vi "Write datatype.vi"(8 "error in (no error)":errorcluster, 10 "datatype":string, 11 "Datatype group in":refnum<class "Datatype group.lvclass">) -> (0 "error out":errorcluster, 3 "Datatype group out":refnum<class "Datatype group.lvclass">)   [LabVIEW 2016, in "FPGA RM Shared API.lvlib" / "Datatype group.lvclass"]
uses:
  Datatype group.lvclass
  Datatype group.lvclass/Datatype group.ctl
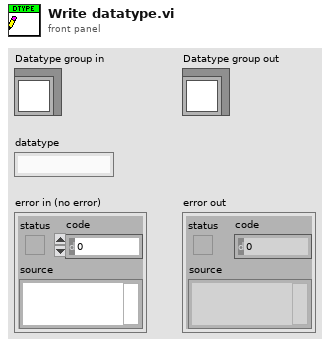
[diagram p1: front panel]
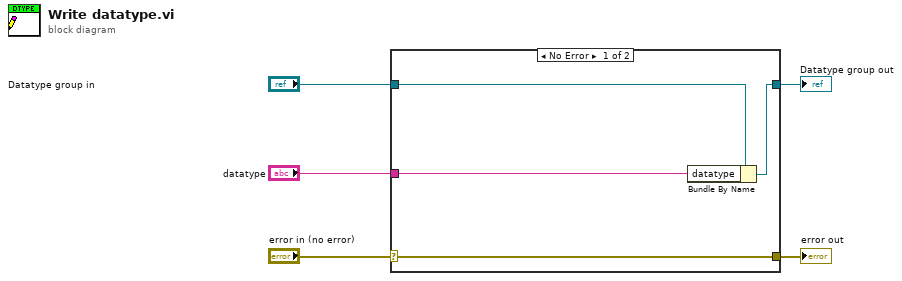
[diagram p0: block diagram]
diagram:
  n1 = case shown="No Error" "error in (no error)" {
    selector: "error in (no error)" -> [w9 w10]
    tunnel: [w9 w10] -> w4
    tunnel: [w7 w11] -> w2
    tunnel: "Datatype group in" -> [w8 w11]
    tunnel: "datatype" -> [w6 _]
    frame No Error {
      n2 = Bundle By Name(cluster=w8, "datatype"=w6) -> (w7:refnum<class "Datatype group.lvclass">)
    }
    frame Error {
    }
  }
  "error out" <- w4
  "Datatype group out" <- w2
